vi "Update tolerance settings.vi"(8 "error in (no error)":errorcluster, 10 "Select a part":refnum<vi>, 11 "ZenGage v3.0 UI in":refnum<class "ZenGage v3.0 UI.lvclass">) -> (0 "error out":errorcluster, 3 "ZenGage v3.0 UI out":refnum<class "ZenGage v3.0 UI.lvclass">)   [LabVIEW 2015, in "ZenGage v3.0 UI.lvclass"]
uses:
  ZenGage v3.0 UI.lvclass
  Type Definitions/General/UI States(UI button enable disable).ctl
  ZenGage v3.0 UI.lvclass/ZenGage v3.0 UI.ctl
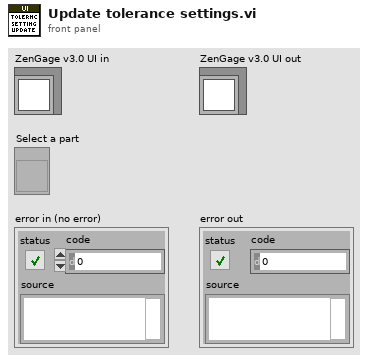
[diagram p1: front panel]
types:
  T1 = typedef "ZenGage v3.0 UI.lvclass/UI States(UI button enable disable).ctl" = cluster{"Inspection":cluster{"Inspection States":enum16{"PreSelect", "Back _Inspection", "Analytics", "Ready To Run", "Ready To Insert", "Enable All buttons", "Disable All Buttons", "Settings", "Select", "Stop", "Pause", "Inspect"}}, "Diagnostics":cluster{"Diagnostics States":enum16{"Enable All", "Camera Optics Fail", "Loading Bar", "Camera Optics", "Motor", "Arduino", "POST Done", "POST"}}, "Edit Tolerance":cluster{"Edit Limits":enum16{"Update List"}, "Enable Disable Measurements":enum16{"Back to Edit Tolerance"}, "Page Select":enum16{"Edit Tolerance Limits", "Enable Disable Buttons"}}, "Page Select":enum16{"Edit Tolerance", "Diagnostics", "Inspection"}}
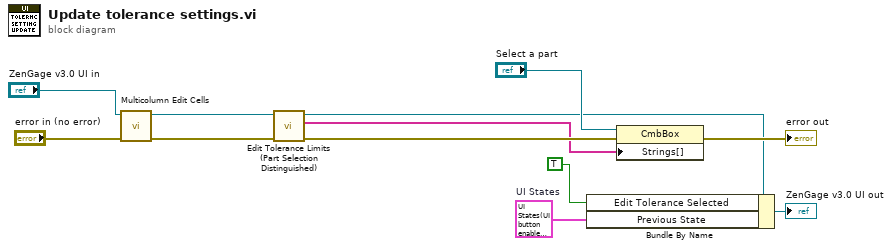
[diagram p0: block diagram]
diagram:
  w6 = T1 {"Inspection"={"Inspection States"=enum."Back _Inspection"}, "Diagnostics"={"Diagnostics States"=enum."Enable All"}, "Edit Tolerance"={"Edit Limits"=enum."Update List", "Enable Disable Measurements"=enum."Back to Edit Tolerance", "Page Select"=enum."Edit Tolerance Limits"}, "Page Select"=enum."Edit Tolerance"}  # UI States
  n1 = call-dynamic "Multicolumn Edit Cells.vi"("error in (no error)"="error in (no error)", "ZenGage v3.0 UI in"="ZenGage v3.0 UI in") -> ("error out"=w8:errorcluster, "ZenGage v3.0 UI out"=w5:refnum<class "ZenGage v3.0 UI.lvclass">)  [unwired: 8 in]
  n2 = call "Edit Tolerance Limits (Part Selection Distinguished).vi"("error in (no error)"=w8, "ZenGage v3.0 UI in"=w5) -> ("error out"=w9:errorcluster, "Parts List out"=w4:string[], "ZenGage v3.0 UI out"=w3:refnum<class "ZenGage v3.0 UI.lvclass">)  [unwired: 7 in]
  n3 = Bundle By Name(cluster=w3, "Edit Tolerance Selected"=TRUE ("General.Edit Tolerance Selected"), "Previous State"=w6) -> (→"ZenGage v3.0 UI out":refnum<class "ZenGage v3.0 UI.lvclass">)
  n4 = property class="CmbBox"(reference="Select a part", error in=w9, "Strings[]"=w4) -> (error out=→"error out":errorcluster)  [unwired: 1 out]
